vi "Using Temperature.vi"() -> ()   [LabVIEW 2014]
panel:
  in  "停止按钮":bool
  out "温度图表":dbl(graph)
  in  "延迟乘数":dbl(knob)=1.0 min=0.0 max=2.0 step=0.1 scale=0.0..2.0
  in  "测量次数":i32=100
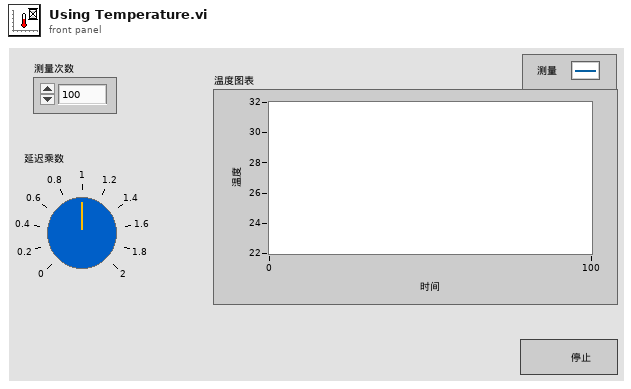
[diagram p1: front panel]
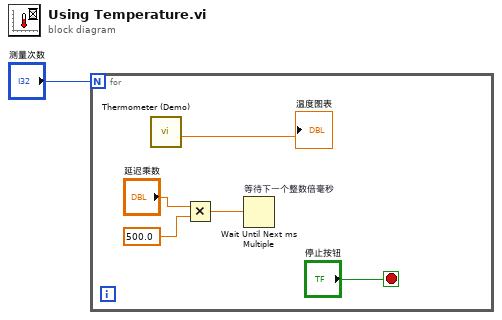
[diagram p0: block diagram]
diagram:
  n1 = for {
    N: "测量次数" -> [_]
    stop <- "停止按钮" stop-if-true
    n2 = call "Thermometer (Demo).vi"() -> ("温度值"=→"温度图表":dbl)  [unwired: 11 in]
    n3 = Multiply(x="延迟乘数", y=500.0) -> (x*y=w4:dbl)
    n4 = Wait Until Next ms Multiple "等待下一个整数倍毫秒"(millisecond multiple=w4) -> ()  [unwired: 1 out]
  }
